vi "send_SQMS_msg_LCW.vi"(5 "alarm_interval":dbl=300.0, 6 "msg":string="https://e906-gat1.fnal.gov/data-summary/e1039/target-LCW.php", 7 "enabled":bool=TRUE, 8 "time_last_alarm_in":timestamp, 9 "title":string="Roots-Pump LCW Flow", 10 "warning":bool, 11 "error":bool) -> (0 "time_last_alarm_out":timestamp, 3 "alarm_status":u32(colorbox), 4 "msg_status":bool)   [LabVIEW 2019]
panel:
  out "full_message":string
  out "resp2":string
  out "resp1":string
  out "resp3":string
  in  "timeout":i32=1000
  in  "port":u16=11111
  in  "address":string="192.168.24.72"
  # "\"time_..._in\" and \"time_..._out\" must be connected\n via Feedback Node or Shift Register in a loop that calls this sub VI."
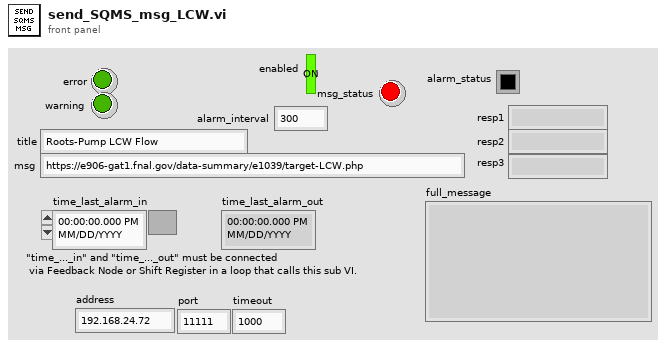
[diagram p1: front panel]
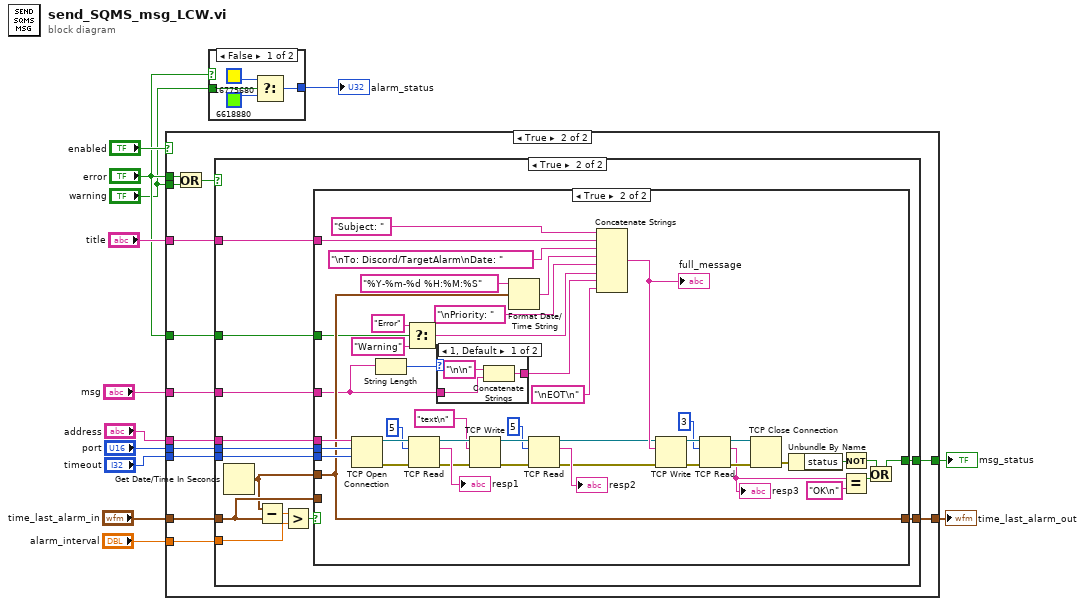
[diagram p0: block diagram]
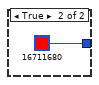
[diagram p2: hidden frame]
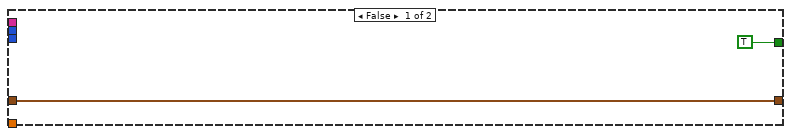
[diagram p3: hidden frame]
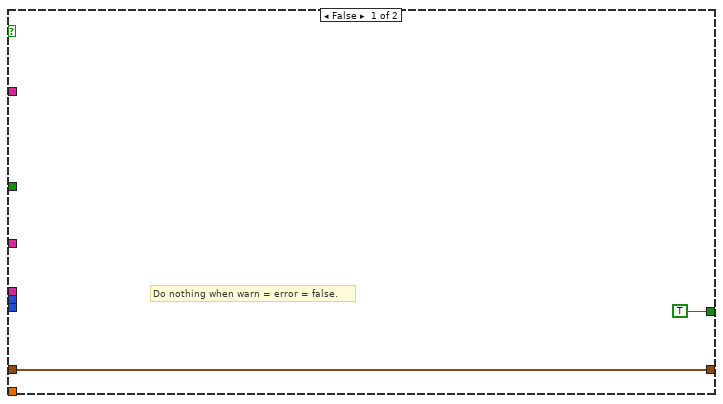
[diagram p4: hidden frame]
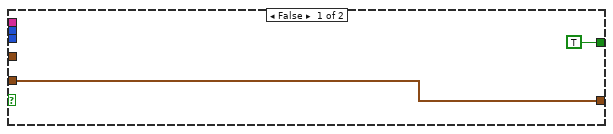
[diagram p5: hidden frame]
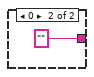
[diagram p6: hidden frame]
diagram:
  n1 = case shown="True" "enabled" {
    tunnel: "error" -> [_ w28]
    tunnel: "warning" -> [_ w27]
    tunnel: [w15 w25] -> w12
    tunnel: "time_last_alarm_in" -> [w15 w24]
    tunnel: "alarm_interval" -> [_ w23]
    tunnel: "address" -> [_ w22]
    tunnel: "port" -> [_ w21]
    tunnel: "timeout" -> [_ w20]
    tunnel: "title" -> [_ w19]
    tunnel: "error" -> [_ w18]
    tunnel: [TRUE w17] -> w5
    tunnel: "msg" -> [_ w16]
    frame False {
    }
    frame True {
      n2 = Or(x=w28, y=w27) -> (x .or. y?=w26:bool)
      n3 = case shown="True" w26 {
        tunnel: [w30 w40] -> w25
        tunnel: w24 -> [w30 w39]
        tunnel: w23 -> [_ w42]
        tunnel: w22 -> [_ w37]
        tunnel: w21 -> [_ w36]
        tunnel: w20 -> [_ w35]
        tunnel: w19 -> [_ w34]
        tunnel: w18 -> [_ w33]
        tunnel: [TRUE w32] -> w17
        tunnel: w16 -> [_ w31]
        frame False {
          # "Do nothing when warn = error = false."
        }
        frame True {
          n4 = Get Date/Time In Seconds() -> (seconds since 1Jan1904=w38:timestamp)
          n5 = Subtract(x=w38, y=w39) -> (x-y=w43:dbl)
          n6 = Greater?(x=w43, y=w42) -> (0:w41:bool)
          n7 = case shown="True" w41 {
            tunnel: [w45 w81] -> w40
            tunnel: w39 -> [w45 _]
            tunnel: w38 -> [_ w81]
            tunnel: w37 -> [_ w89]
            tunnel: w36 -> [_ w88]
            tunnel: w35 -> [_ w87]
            tunnel: w34 -> [_ w84]
            tunnel: w33 -> [_ w73]
            tunnel: [TRUE w50] -> w32
            tunnel: w31 -> [_ w46]
            frame False {
            }
            frame True {
              n8 = TCP Open Connection(address=w89, remote port or service name=w88, timeout ms (60000)=w87) -> (connection ID=w86:refnum<k5>, error out=w60:errorcluster)  [unwired: 2 in]
              n9 = String Length(string=w46) -> (length=w48:i32)
              n10 = Select(t="Error", s=w73, f="Warning") -> (s? t:f=w71:string)
              n11 = TCP Read(connection ID=w86, bytes to read=5, error in (no error)=w60) -> (connection ID out=w68:refnum<k5>, data out=→"resp1":string, error out=w59:errorcluster)  [unwired: 2 in]
              n12 = case shown="1, Default" w48 {
                tunnel: [w92 ""] -> w47
                tunnel: w46 -> [w90 _]
                frame 1, Default {
                  n13 = Concatenate Strings("\n\n" ("string"), w90) -> (w92:string)
                }
                frame 0 {
                }
              }
              n14 = TCP Write(connection ID=w68, data in="text\n", error in (no error)=w59) -> (connection ID out=w65:refnum<k5>, error out=w58:errorcluster)  [unwired: 1 in, 1 out]
              n15 = Format Date/Time String(time format string (%c)="%Y-%m-%d %H:%M:%S", seconds (now)=w81) -> (date/time string=w80:string)  [unwired: 1 in]
              n16 = TCP Read(connection ID=w65, bytes to read=5, error in (no error)=w58) -> (connection ID out=w63:refnum<k5>, data out=→"resp2":string, error out=w57:errorcluster)  [unwired: 2 in]
              n17 = Concatenate Strings("Subject: ", w84, "\nTo: Discord/TargetAlarm\nDate: ", w80, "\nPriority: ", w71, w47, "\nEOT\n") -> (w78:string)
              "full_message" <- w78
              n18 = TCP Write(connection ID=w63, data in=w78, error in (no error)=w57) -> (connection ID out=w77:refnum<k5>, error out=w76:errorcluster)  [unwired: 1 in, 1 out]
              n19 = TCP Read(connection ID=w77, bytes to read=3, error in (no error)=w76) -> (connection ID out=w74:refnum<k5>, data out=w54:string, error out=w75:errorcluster)  [unwired: 2 in]
              "resp3" <- w54
              n20 = TCP Close Connection(connection ID=w74, error in (no error)=w75) -> (error out=w56:errorcluster)  [unwired: 1 in, 1 out]
              n21 = Unbundle By Name(w56) -> ("status"=w55:bool)
              n22 = Not(x=w55) -> (.not. x?=w51:bool)
              n23 = Equal?(x=w54, y="OK\n") -> (x = y?=w52:bool)
              n24 = Or(x=w51, y=w52) -> (x .or. y?=w50:bool)
            }
          }
        }
      }
    }
  }
  "time_last_alarm_out" <- w12
  "msg_status" <- w5
  n25 = case shown="False" "error" {
    tunnel: "warning" -> [w97 _]
    tunnel: [w94 u32 16711680 ("alarm_status")] -> w1
    frame False {
      n26 = Select(t=u32 16775680 ("alarm_status"), s=w97, f=u32 6618880 ("alarm_status")) -> (s? t:f=w94:u32)
    }
    frame True {
    }
  }
  "alarm_status" <- w1
